vi "Generate Overlap SQL Query.vi"(8 "error in (no error)":errorcluster, 10 "num of csv transactions":i32, 11 "Transaction in":refnum<class "Transaction.lvclass">) -> (0 "error out":errorcluster, 2 "SQL Query":string, 3 "Transaction out":refnum<class "Transaction.lvclass">)   [LabVIEW 2018, in "Transaction.lvclass"]
uses:
  Transaction.lvclass
  Transaction.lvclass/Transaction.ctl
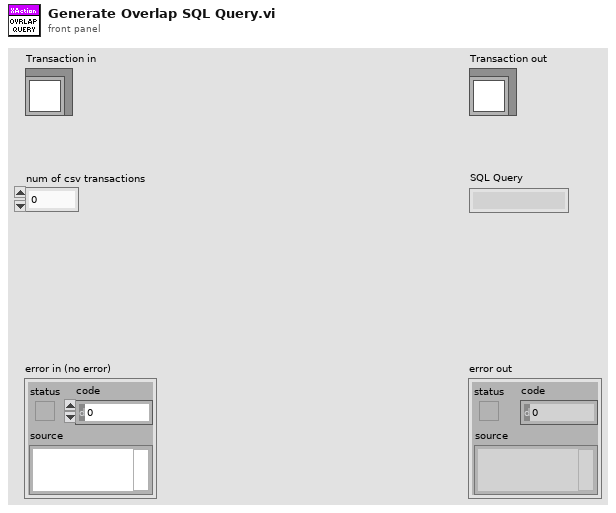
[diagram p1: front panel]
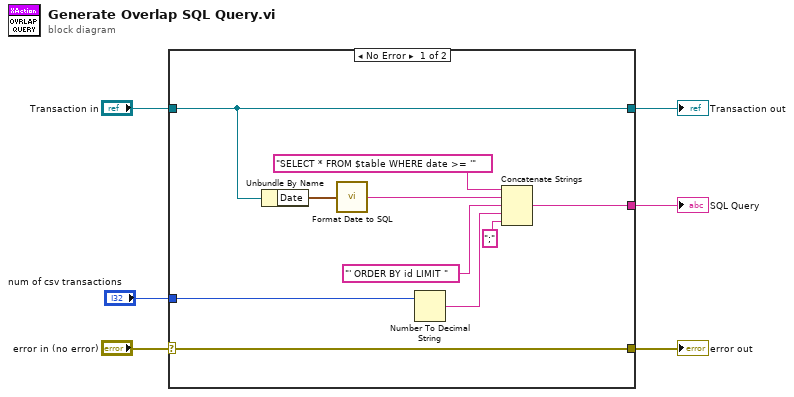
[diagram p0: block diagram]
diagram:
  n1 = case shown="No Error" "error in (no error)" {
    selector: "error in (no error)" -> [w16 w18]
    tunnel: [w16 w18] -> w5
    tunnel: [w15 w17] -> w3
    tunnel: "Transaction in" -> [w15 w17]
    tunnel: "num of csv transactions" -> [w8 _]
    tunnel: [w7 _] -> w1
    frame No Error {
      n2 = Unbundle By Name(w15) -> ("Date"=w14:timestamp)
      n3 = call "Format Date to SQL.vi"("Date"=w14) -> ("SQL Date"=w9:string)
      n4 = Number To Decimal String(number=w8) -> (decimal integer string=w11:string)  [unwired: 1 in]
      n5 = Concatenate Strings("SELECT * FROM $table WHERE date >= '", w9, "' ORDER BY id LIMIT " ("string"), w11, ";" ("string")) -> (w7:string)
    }
    frame Error {
    }
  }
  "error out" <- w5
  "Transaction out" <- w3
  "SQL Query" <- w1
